vi "Strip Path To Exe.vi"(11 "VI Path":path) -> (1 "Found exe?":bool, 2 "exe Name":string, 3 "exe Dir":path)   [LabVIEW 2019, in "LMH-Toolbox.lvlib"]
doc: "This VI returns the abolute path up to the '.exe' token. This VI can be used to find the path of a LabVIEW built exe on disk by passing the callers path as the VI Path input."
uses:
  <vilib>/MakerHub/Toolbox/LMH-Toolbox.lvlib
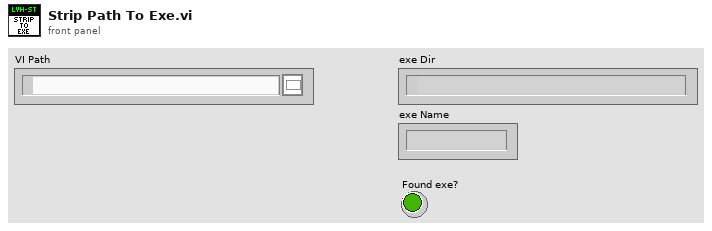
[diagram p1: front panel]
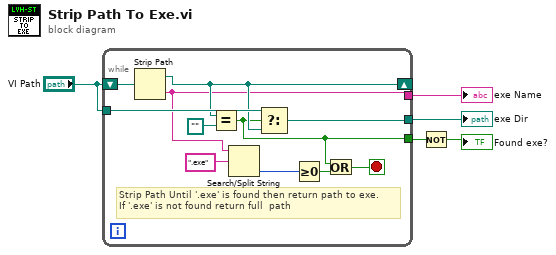
[diagram p0: block diagram]
diagram:
  n1 = while {
    shift-right: [w9] -> _
    shift-left: "VI Path" -> [w16]
    tunnel: "VI Path" -> [w10]
    tunnel: [w8] -> w4
    tunnel: [w7] -> w3
    tunnel: [w6] -> w1
    stop <- w11 stop-if-true
    # "Strip Path Until '.exe' is found then return path to exe.\nIf '.exe' is not found return full  path"
    n2 = Strip Path(path=w16) -> (stripped path=w9:path, name=w6:string)
    n3 = Equal?(x=w9, y=path "") -> (x = y?=w7:bool)
    n4 = Search/Split String(string=w6, search string/char (-)=".exe") -> (offset of match=w13:i32)  [unwired: 1 in, 2 out]
    n5 = Select(t=w10, s=w7, f=w9) -> (s? t:f=w8:path)
    n6 = Greater Or Equal To 0?(x=w13) -> (x >= 0?=w12:bool)
    n7 = Or(x=w7, y=w12) -> (x .or. y?=w11:bool)
  }
  "exe Dir" <- w4
  "exe Name" <- w1
  n8 = Not(x=w3) -> (.not. x?=→"Found exe?":bool)
